vi "SHA-1myString.vi"(10 "HashThis":string) -> (1 "SHAdata":u8[](array[numeric]) format="%.0x", 2 "SHA1string":string)   [LabVIEW 2022 SP3]
panel:
  # "Obtained from: https://decibel.ni.com/content/docs/DOC-10292"
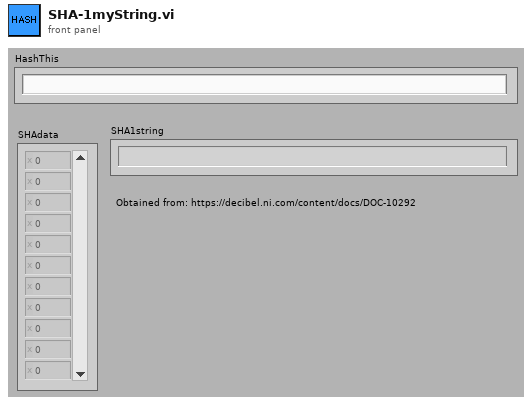
[diagram p1: front panel]
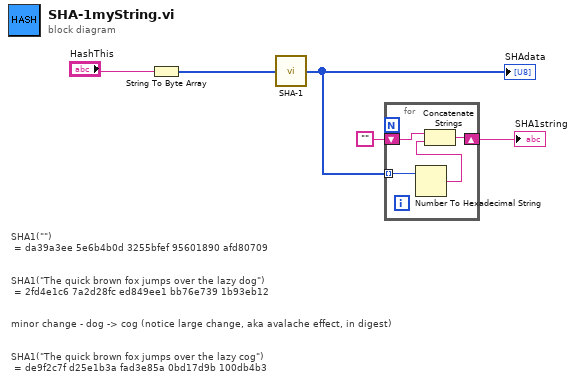
[diagram p0: block diagram]
diagram:
  # "minor change - dog -> cog (notice large change, aka avalache effect, in digest)"
  # "SHA1(\"The quick brown fox jumps over the lazy dog\") \n = 2fd4e1c6 7a2d28fc ed849ee1 bb76e739 1b93eb12"
  # "SHA1(\"The quick brown fox jumps over the lazy cog\") \n = de9f2c7f d25e1b3a fad3e85a 0bd17d9b 100db4b3"
  # "SHA1(\"\")\n = da39a3ee 5e6b4b0d 3255bfef 95601890 afd80709"
  n1 = String To Byte Array(string="HashThis") -> (unsigned byte array=w5:u8[])
  n2 = call "SHA-1.vi"("Data"=w5) -> ("message-digest"=w1:u8[])
  "SHAdata" <- w1
  n3 = for {
    tunnel: w1 -> [w9] mode=indexing
    shift-right: [w7] -> w2
    shift-left: "" -> [w8]
    n4 = Number To Hexadecimal String(2:w9) -> (0:w6:string)  [unwired: 1 in]
    n5 = Concatenate Strings(w8, w6) -> (w7:string)
  }
  "SHA1string" <- w2
